vi "ArmChange.vi"(11 "refnum name":string) -> ()   [LabVIEW 2019]
uses:
  <vilib>/Rock Robotics/WPI/SafetyOutput/WPI_SafetyOutputConfigMenu.ctl
  <vilib>/Rock Robotics/SystemInterfaces/DIO/FPGA_DIOChannel.ctl
  <vilib>/Rock Robotics/WPI/RobotDrive/WPI_RobotDriveOpen2MotorWithExistingMotors.vi
  <vilib>/Rock Robotics/WPI/Switch/WPI_SwitchOpenLimit.vi
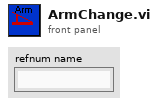
[diagram p1: front panel]
types:
  T1 = typedef "FPGA_DIOChannel.ctl" = enum8{"DIO 0", "DIO 1", "DIO 2", "DIO 3", "DIO 4", "DIO 5", "DIO 6", "DIO 7", "DIO 8", "DIO 9", "DIO MXP 0", "DIO MXP 1", "DIO MXP 2", "DIO MXP 3", "DIO MXP 4", "DIO MXP 5", "DIO MXP 6", "DIO MXP 7", "DIO MXP 8", "DIO MXP 9", "DIO MXP 10", "DIO MXP 11", "DIO MXP 12", "DIO MXP 13", "DIO MXP 14", "DIO MXP 15", "SPI Port CS1", "SPI Port CS2", "SPI Port CS3", "SPI Port MISO", "SPI Port MOSI", "Invalid"}
  T2 = typedef "WPI_SafetyOutputConfigMenu.ctl" = enum16{"Enable", "Disable"}
  T3 = typedef "WPI_MotorControlDeviceRef.ctl" = cluster{"DeviceStatus":errorcluster, "Type":T4, "PWM":cluster{"PWM Channel":T5, "DeadBand":T6}, "CAN":cluster{"Device Number":u8, "SetOutput VI Ref":variant, "GetOutput VI Ref":variant, "Enable VI Ref":variant, "Disable VI Ref":variant, "Data":variant}, "Invert":bool, "DIO PWM":cluster{"PWM \"Enable\" Channel":T5, "DIOChannel":T1, "PWM Rate":dbl}}
  T4 = typedef "WPI_MotorControlType.ctl" = enum16{"PWM", "CAN", "DIO PWM"}
  T5 = typedef "FPGA_DIOPWMChannel.ctl" = enum8{"PWM 0", "PWM 1", "PWM 2", "PWM 3", "PWM 4", "PWM 5", "PWM 6", "PWM 7", "PWM 8", "PWM 9", "PWM MXP 0", "PWM MXP 1", "PWM MXP 2", "PWM MXP 3", "PWM MXP 4", "PWM MXP 5", "PWM MXP 6", "PWM MXP 7", "PWM MXP 8", "PWM MXP 9", "Invalid"}
  T6 = typedef "WPI_PWMDeadband.ctl" = cluster{"Name":string, "maxPositivePwm":i32, "minPositivePwm":i32, "centerPwm":i32, "maxNegativePwm":i32, "minNegativePwm":i32, "angularRange":u16}
  T7 = typedef "WPI_RobotDriveDevRef.ctl" = cluster{"DevStatus":errorcluster, "Motors[]":T3[], "Square Inputs":bool, "Max Output":dbl}
  T8 = typedef "WPI_SwitchDevRef.ctl" = cluster{"DevStatus":errorcluster, "DIO Channel":T1, "CntIndex":T9, "Normally Closed":bool}
  T9 = typedef "FPGA_CounterCtrSystemIndex.ctl" = enum8{"Ctr 0", "Ctr 1", "Ctr 2", "Ctr 3", "Ctr 4", "Ctr 5", "Ctr 6", "Ctr 7", "Invalid"}
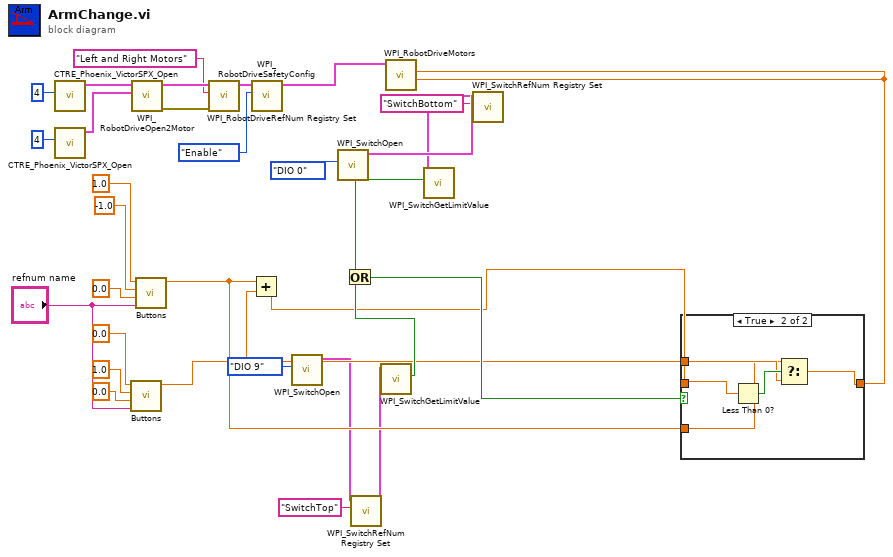
[diagram p0: block diagram]
diagram:
  n1 = call <vilib>:"CTRE_Phoenix_VictorSPX_Open.vi"("Device Number"=u8 4) -> ("CAN Talon SRX Ref"=w21:T3)  [unwired: 9 in, 1 out]
  n2 = call <vilib>:"CTRE_Phoenix_VictorSPX_Open.vi"("Device Number"=u8 4) -> ("CAN Talon SRX Ref"=w23:T3)  [unwired: 9 in, 1 out]
  n3 = call "Buttons.vi"("Joystick Name"="refnum name", "Button Not Pressed Speed"=0.0, "Button Pressed Speed"=1.0, "Button Index"=0.0) -> ("Numeric"=w7:dbl)  [unwired: 7 in]
  n4 = call-poly <vilib>:"WPI_RobotDriveOpen2Motor.vi"("Right Motor Dev Ref"=w23, "Left Motor Dev Ref"=w21) -> ("error out"=w24:errorcluster, "RobotDriveDevRef"=w19:T7)  [unwired: 8 in]
  n5 = call "Buttons.vi"("Joystick Name"="refnum name", "Button Not Pressed Speed"=0.0, "Button Pressed Speed"=-1.0, "Button Index"=1.0) -> ("Numeric"=w8:dbl)  [unwired: 7 in]
  n6 = call <vilib>:"WPI_RobotDriveRefNum Registry Set.vi"("error in (no error)"=w24, "refnum name"="Left and Right Motors", "RobotDriveDevRef"=w19) -> ("RobotDriveDevRef"=w17:T7)  [unwired: 1 in, 7 out]
  n7 = Add(x=w8, y=w7) -> (x+y=w10:dbl)
  n8 = call <vilib>:"WPI_RobotDriveSafetyConfig.vi"("mode"=WPI_SafetyOutputConfigMenu."Enable", "RobotDriveDevRef"=w17) -> ("RobotDriveDevRef"=w31:T7)  [unwired: 8 in, 1 out]
  n9 = call-poly <vilib>:"WPI_SwitchOpen.vi"("DIO Channel"=FPGA_DIOChannel."DIO 9") -> ("SwitchDevRef"=w6:T8)  [unwired: 9 in, 1 out]
  n10 = call-poly <vilib>:"WPI_SwitchOpen.vi"("DIO Channel"=FPGA_DIOChannel."DIO 0") -> ("SwitchDevRef"=w4:T8)  [unwired: 9 in, 1 out]
  n11 = call <vilib>:"WPI_SwitchRefNum Registry Set.vi"("refnum name"="SwitchTop", "SwitchDevRef"=w6) -> ("SwitchDevRef"=w5:T8)  [unwired: 8 in, 1 out]
  n12 = call <vilib>:"WPI_SwitchGetLimitValue.vi"("SwitchDevRef"=w5) -> ("Switch Pressed"=w12:bool)  [unwired: 8 in, 2 out]
  n13 = call <vilib>:"WPI_SwitchRefNum Registry Set.vi"("refnum name"="SwitchBottom", "SwitchDevRef"=w4) -> ("SwitchDevRef"=w3:T8)  [unwired: 8 in, 1 out]
  n14 = call <vilib>:"WPI_SwitchGetLimitValue.vi"("SwitchDevRef"=w3) -> ("Switch Pressed"=w13:bool)  [unwired: 8 in, 2 out]
  n15 = Or(x=w13, y=w12) -> (x .or. y?=w11:bool)
  n16 = case shown="True" w11 {
    tunnel: [w33 w36] -> w9
    tunnel: w10 -> [w33 w38]
    tunnel: w8 -> [_ w34]
    tunnel: w7 -> [_ w35]
    frame False {
    }
    frame True {
      n17 = Less Than 0?(x=w38) -> (x < 0?=w37:bool)
      n18 = Select(t=w34, s=w37, f=w35) -> (s? t:f=w36:dbl)
    }
  }
  n19 = call <vilib>:"WPI_RobotDriveMotors.vi"("RightSpeed"=w9, "LeftSpeed"=w9, "RobotDriveDevRef"=w31) -> ()  [unwired: 1 in, 8 out]
